vi "HaltSkill.vi"(8 "error in (no error)":errorcluster, 10 "Robot":refnum<class "Robot.lvclass">, 11 "HaltSkill in":refnum<class "HaltSkill.lvclass">) -> (0 "error out":errorcluster, 2 "Robot out":refnum<class "Robot.lvclass">, 3 "HaltSkill out":refnum<class "HaltSkill.lvclass">)   [LabVIEW 2018, in "HaltSkill.lvclass"]
uses:
  HaltSkill.lvclass
  Robot_class/Robot.lvclass
  Robot_class/Robot.lvclass/Robot.ctl
  Robot_class/Write v_tang.vi
  Robot_class/Write v_norm.vi
  Robot_class/Write v_ang.vi
  Robot_class/Write kick_z.vi
  Robot_class/Write kick_x.vi
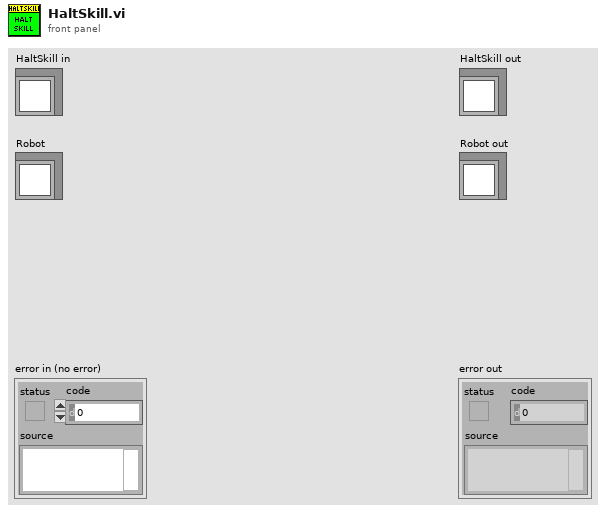
[diagram p1: front panel]
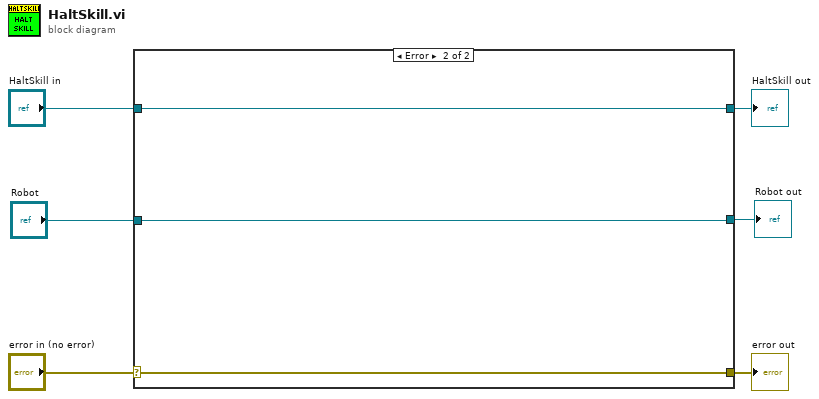
[diagram p0: block diagram]
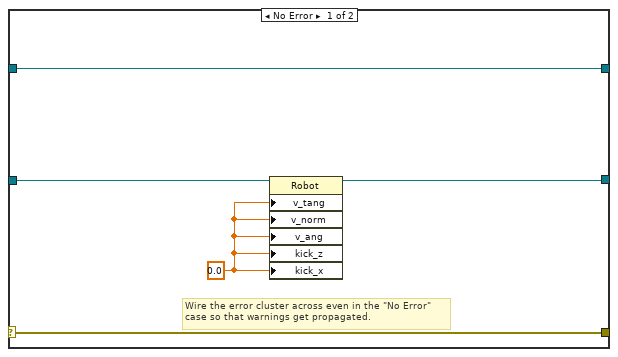
[diagram p2: hidden frame]
diagram:
  n1 = case shown="Error" "error in (no error)" {
    selector: "error in (no error)" -> [w10 w14]
    tunnel: [w10 w14] -> w5
    tunnel: [w11 w13] -> w3
    tunnel: "HaltSkill in" -> [w11 w13]
    tunnel: "Robot" -> [w9 w12]
    tunnel: [w8 w12] -> w1
    frame No Error {
      w7 = 0.0 ("kick_x")
      # "Wire the error cluster across even in the \"No Error\"\ncase so that warnings get propagated."
      n2 = property class="Robot"(reference=w9, "v_tang"=w7, "v_norm"=w7, "v_ang"=w7, "kick_z"=w7, "kick_x"=w7) -> (reference out=w8:refnum<class "Robot.lvclass">)  [unwired: 1 in, 1 out]
    }
    frame Error {
    }
  }
  "error out" <- w5
  "HaltSkill out" <- w3
  "Robot out" <- w1
